vi "Test ICL running.vi"(8 "error in (no error)":errorcluster) -> (0 "error out":errorcluster, 2 "StdErr":string, 3 "icl.exe found":bool)   [LabVIEW 2023]
uses:
  <vilib>/JKI/JKI DotNet System Exec/dotnet_system_exec/dotnet_system_exec.lvclass
panel:
  out "StdOut":string
  # "Connector Pane"
  # "Locals"
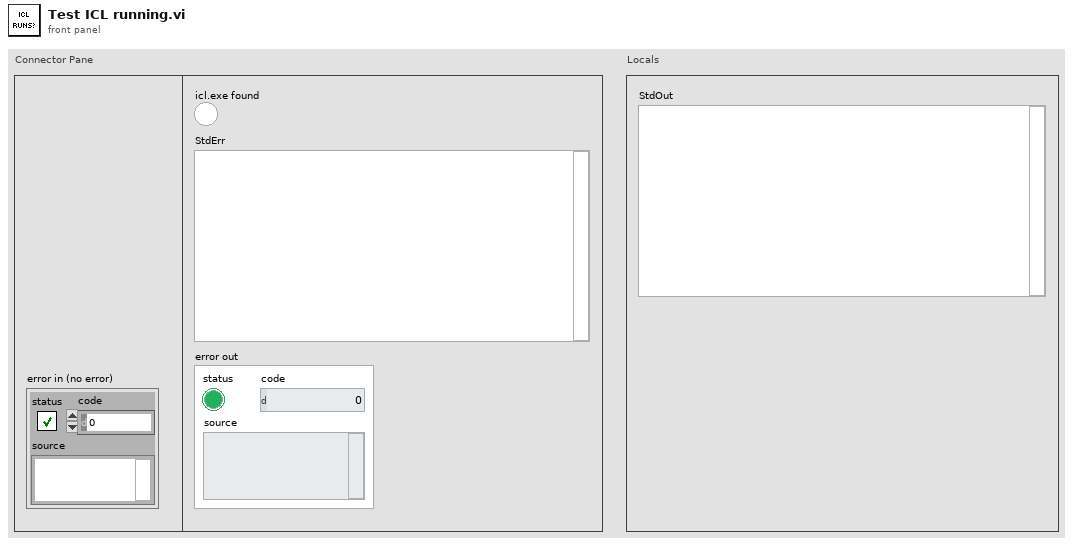
[diagram p1: front panel]
types:
  T1 = cluster{"stdout event":refnum<user-event>, "stderr event":refnum<user-event>, "process_exit event":refnum<user-event>}
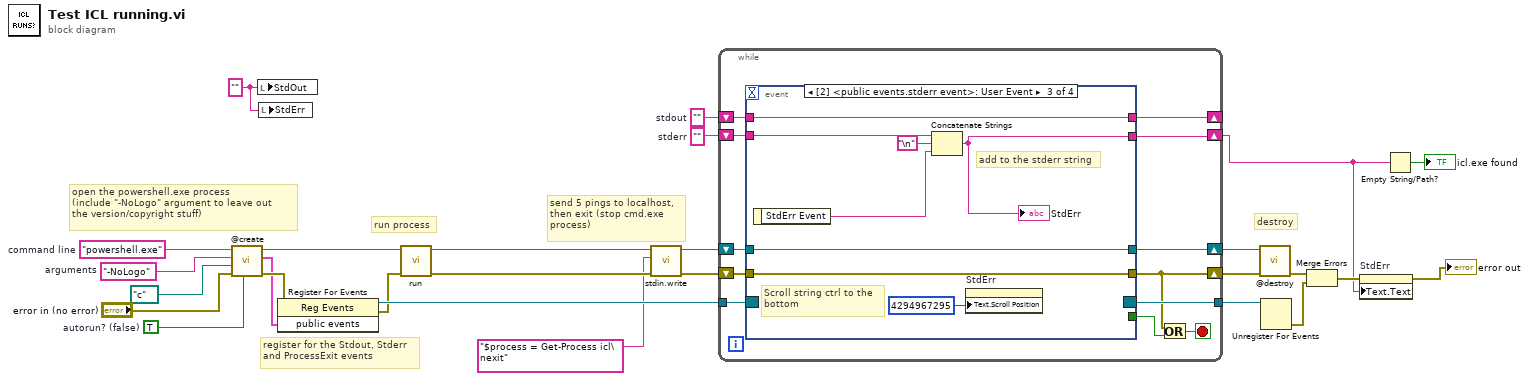
[diagram p0: block diagram]
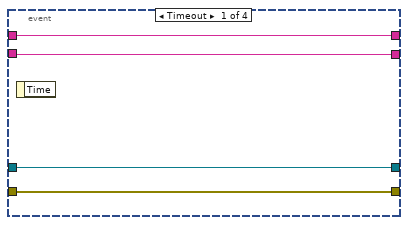
[diagram p2: hidden frame]
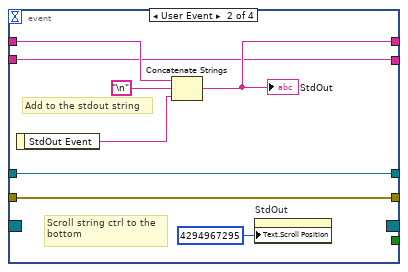
[diagram p3: hidden frame]
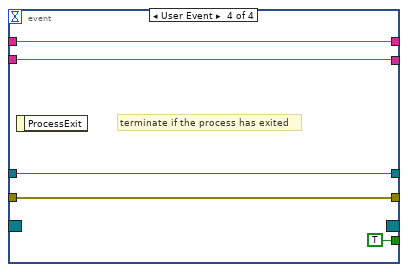
[diagram p4: hidden frame]
diagram:
  w11 = TRUE  # autorun? (false)
  w12 = "" ("Process File Name")
  w14 = ""  # stderr
  w18 = "-NoLogo"  # arguments
  w19 = ""  # stdout
  w20 = "powershell.exe"  # command line
  # "send 5 pings to localhost,\nthen exit (stop cmd.exe \nprocess)"
  # "destroy"
  # "register for the Stdout, Stderr \nand ProcessExit events"
  # "run process"
  # "open the powershell.exe process\n(include \"-NoLogo\" argument to leave out\nthe version/copyright stuff)"
  n1 = call <vilib>:"@create.vi"("autorun? (false)"=w11, "error in (no error)"="error in (no error)", "working directory (c:\\)"=path "c:/" ("working directory"), "arguments (\"\")"=w18, "command line (cmd.exe)"=w20) -> ("error out"=w17:errorcluster, "public events"=w15:T1, "dotnet_system_exec out"=w26:refnum<class "dotnet_system_exec.lvclass">)  [unwired: 4 in]
  n2 = local write "StdOut"(w12) -> ()
  n3 = local write "StdErr"(w12) -> ()
  n4 = register-events(error in=w17, w15) -> (reference out=w25:refnum<event-registration>, error out=w16:errorcluster)  [unwired: 1 in]
  n5 = call <vilib>:"run.vi"("error in (no error)"=w16, "dotnet_system_exec in"=w26) -> ("error out"=w9:errorcluster, "dotnet_system_exec out"=w10:refnum<class "dotnet_system_exec.lvclass">)  [unwired: 8 in]
  n6 = call-dynamic "stdin.write.vi"("error in (no error)"=w9, "stdin"="$process = Get-Process icl\nexit", "dotnet_system_exec in"=w10) -> ("error out"=w7:errorcluster, "dotnet_system_exec out"=w8:refnum<class "dotnet_system_exec.lvclass">)  [unwired: 7 in]
  n7 = while {
    shift-right: [w39] -> w27
    shift-left: w8 -> [w38]
    shift-right: [w30] -> w23
    shift-left: w7 -> [w37]
    tunnel: w25 -> [w36]
    tunnel: [w35] -> w24
    shift-right: [w33] -> _
    shift-left: w19 -> [w34]
    shift-right: [w31] -> w1
    shift-left: w14 -> [w32]
    stop <- w29 stop-if-true
    n8 = event shown="[2] <public events.stderr event>: User Event" {
      selector: w36 -> [_ _ _ _]
      dyn-events: [_ _ _ _] -> w35
      timeout: _ -> [_ _ _ _]
      tunnel: [w43 w51 w59 w62] -> w39
      tunnel: w38 -> [w43 w51 w59 w62]
      tunnel: w37 -> [w42 w50 w58 w61]
      tunnel: [w42 w50 w58 w61] -> w30
      tunnel: w34 -> [w41 w47 w54 w63]
      tunnel: [w41 w48 w54 w63] -> w33
      tunnel: [_ _ _ TRUE ("ProcessExit")] -> w28
      tunnel: w32 -> [w40 w45 w55 w64]
      tunnel: [w40 w45 w53 w64] -> w31
      event Timeout {
        n9 = event-data() -> ()  [unwired: 1 in, 1 out]
      }
      event User Event {
        # "Scroll string ctrl to the \nbottom"
        # "Add to the stdout string"
        n10 = event-data() -> ("StdOut Event"=w46:string)  [unwired: 1 in]
        n11 = Concatenate Strings(w47, "\n", w46) -> (w48:string)
        "StdOut" <- w48
        n12 = property on="StdOut" class="Str"("Text.Scroll Position"=u32 4294967295) -> ()  [unwired: 2 in, 2 out]
      }
      event User Event {
        # "Scroll string ctrl to the \nbottom"
        # "add to the stderr string"
        n13 = event-data() -> ("StdErr Event"=w56:string)  [unwired: 1 in]
        n14 = Concatenate Strings(w55, "\n", w56) -> (w53:string)
        "StdErr" <- w53
        n15 = property on="StdErr" class="Str"("Text.Scroll Position"=u32 4294967295) -> ()  [unwired: 2 in, 2 out]
      }
      event User Event {
        # "terminate if the process has exited"
        n16 = event-data() -> ()  [unwired: 1 in, 1 out]
      }
    }
    n17 = Or(x=w30, y=w28) -> (x .or. y?=w29:bool)
  }
  n18 = call-dynamic "@destroy.vi"("error in (no error)"=w23, "dotnet_system_exec in"=w27) -> ("error out"=w22:errorcluster)  [unwired: 8 in, 1 out]
  n19 = Unregister For Events(event registration refnum=w24) -> (error out=w21:errorcluster)  [unwired: 1 in]
  n20 = Merge Errors(w22, w21) -> (w3:errorcluster)
  n21 = property on="StdErr" class="Str"(error in=w3, "Text.Text"=w1) -> (error out=→"error out":errorcluster)  [unwired: 1 in, 1 out]
  n22 = Empty String/Path?(string/path=w1) -> (empty?=→"icl.exe found":bool)
